vi "OpenSink.vi"(8 "error in (no error)":errorcluster, 11 "RelayAppender in":refnum<class "RelayAppender.lvclass">) -> (0 "error out":errorcluster, 3 "RelayAppender out":refnum<class "RelayAppender.lvclass">)   [LabVIEW 2026, in "Lumberjack.lvlib" / "RelayAppender.lvclass"]
doc: "Override of Appender.OpenSink, run once on actor startup. Queue mode: obtains the relay queue by its id-derived name (element type Statement) so the actor shares the same named queue the application holds, and stores the refnum in private data for Write to enqueue into. Message mode: validates the consumer enqueuer. Raises Lumberjack error +26 if the required resource is missing (queue not obtainable, or invalid enqueuer). Protected, dynamic-dispatch."
uses:
  RelayAppender.lvclass
  C:/Users/dallis/OneDrive - Velico Medical/Documents/Personal/LabVIEW Coding Projects/Lumberjack/src/Core/Appenders/Appender.lvclass/Appender.lvclass
  RelayAppender.lvclass/RelayAppender.ctl
  TypeDefs/Statement.ctl
  TypeDefs/Severity.ctl
  <vilib>/ActorFramework/Message Enqueuer/Message Enqueuer.lvclass
  Lumberjack.lvlib
  Appender.lvclass/Appender.lvclass
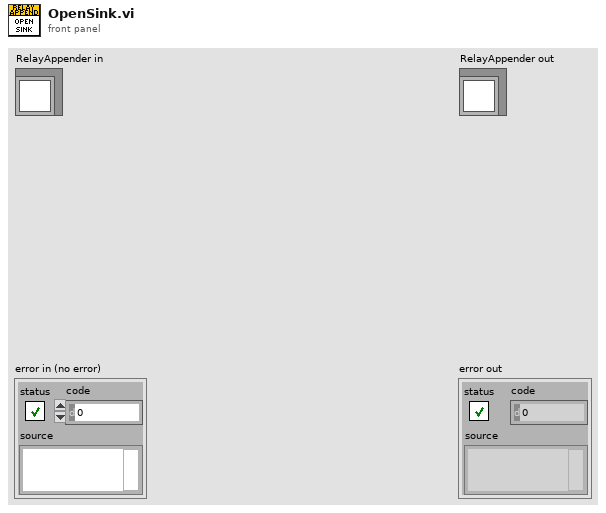
[diagram p1: front panel]
types:
  T1 = typedef "Lumberjack.lvlib/Statement.ctl" = cluster{"timestamp":timestamp, "level":T2, "sourceTag":string, "originVI":string, "message":string}
  T2 = typedef "Lumberjack.lvlib/Severity.ctl" = enum16{"OFF", "FATAL", "ERROR", "WARN", "INFO", "DEBUG", "TRACE", "ALL"}
  T3 = typedef "Lumberjack.lvlib/RelayMode.ctl" = enum16{"Message", "Queue"}
  T4 = typedef "Lumberjack.lvlib/AppenderConfig.ctl" = cluster{"id":string, "threshold":T2, "filter":T5, "queueBound":i32, "dropPolicy":T7, "useUTC":bool}
  T5 = typedef "Lumberjack.lvlib/Filter.ctl" = cluster{"mode":T6, "levelMin":T2, "levelMax":T2, "tagPrefix":string}
  T6 = typedef "Lumberjack.lvlib/FilterMode.ctl" = enum16{"Mirror", "Routed"}
  T7 = typedef "Lumberjack.lvlib/DropPolicy.ctl" = enum16{"DropOldest", "DropNewest", "LevelAware"}
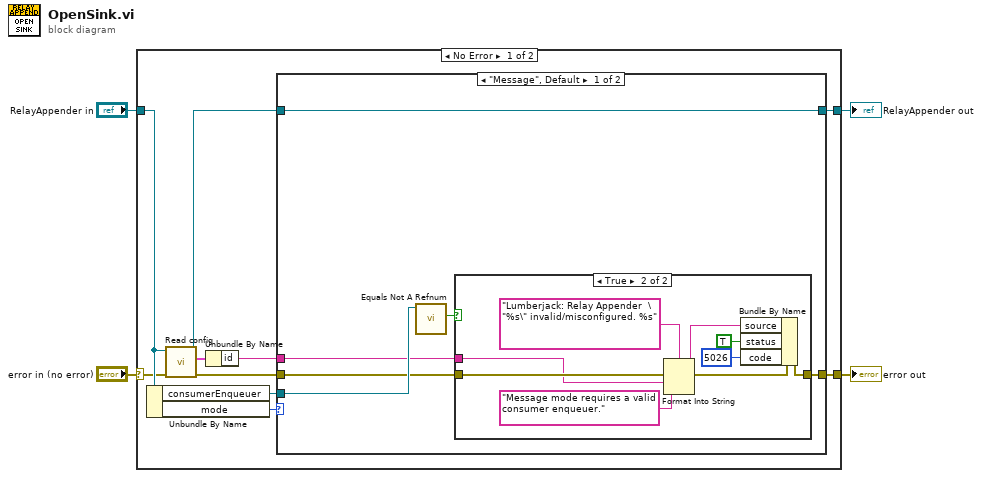
[diagram p0: block diagram]
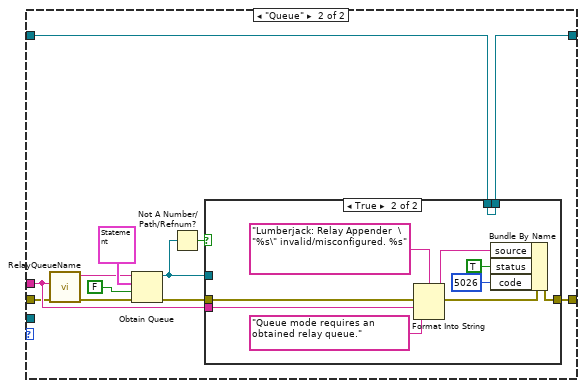
[diagram p3: hidden frame]
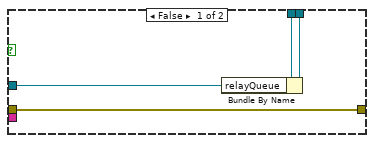
[diagram p4: hidden frame]
diagram:
  n1 = case shown="No Error" "error in (no error)" {
    selector: "error in (no error)" -> [w9 w58]
    tunnel: [w14 w58] -> w4
    tunnel: [w13 w57] -> w3
    tunnel: "RelayAppender in" -> [w10 w57]
    frame No Error {
      n2 = Unbundle By Name(w10) -> ("consumerEnqueuer"=w12:refnum<class "Message Enqueuer.lvclass">, "mode"=w11:T3)
      n3 = call "Read config.vi"("error in (no error)"=w9, "Appender in"=w10) -> ("error out"=w6:errorcluster, "AppenderConfig"=w8:T4, "Appender out"=w5:refnum<class "RelayAppender.lvclass">)  [unwired: 7 in]
      n4 = Unbundle By Name(w8) -> ("id"=w7:string)
      n5 = case shown="\"Message\", Default" w11 {
        tunnel: w12 -> [w20 _]
        tunnel: [w19 w42] -> w14
        tunnel: [w17 w37] -> w13
        tunnel: w7 -> [w15 w33]
        tunnel: w6 -> [w16 w32]
        tunnel: w5 -> [w17 w31]
        frame "Message", Default {
          n6 = call <vilib>:"Equals Not A Refnum.vi"("Message Enqueuer"=w20) -> ("Not a refnum?"=w18:bool)  [unwired: 10 in]
          n7 = case shown="True" w18 {
            tunnel: [w21 w25] -> w19
            tunnel: w16 -> [w21 w26]
            tunnel: w15 -> [_ w23]
            frame False {
            }
            frame True {
              n8 = Format Into String(format string="Lumberjack: Relay Appender  \"%s\" invalid/misconfigured. %s" ("source"), error in=w26, w23, "Message mode requires a valid consumer enqueuer.") -> (resulting string=w30:string, error out=w24:errorcluster)  [unwired: 1 in]
              n9 = Bundle By Name(cluster=w24, "source"=w30, "status"=TRUE, "code"=5026) -> (w25:errorcluster)
            }
          }
        }
        frame "Queue" {
          n10 = call "RelayQueueName.vi"("error in (no error)"=w32, "id"=w33) -> ("error out"=w35:errorcluster, "queueName"=w34:string)  [unwired: 8 in]
          n11 = Obtain Queue(name (unnamed)=w34, element data type=T1 {"timestamp"=timestamp(0 s since 1904-01-01), "level"=enum."INFO", "sourceTag"="", "originVI"="", "message"=""} ("Statement"), create if not found? (T)=FALSE, error in (no error)=w35) -> (queue out=w36:refnum<queue>, error out=w40:errorcluster)  [unwired: 1 in, 1 out]
          n12 = Not A Number/Path/Refnum?(number/path/refnum=w36) -> (NaN/Path/Refnum?=w41:bool)
          n13 = case shown="True" w41 {
            tunnel: [w46 w51] -> w42
            tunnel: w40 -> [w46 w52]
            tunnel: w33 -> [_ w50]
            tunnel: w31 -> [w45 w48]
            tunnel: [w44 w48] -> w37
            tunnel: w36 -> [w43 _]
            frame False {
              n14 = Bundle By Name(cluster=w45, "relayQueue"=w43) -> (w44:refnum<class "RelayAppender.lvclass">)
            }
            frame True {
              n15 = Format Into String(format string="Lumberjack: Relay Appender  \"%s\" invalid/misconfigured. %s" ("source"), error in=w52, w50, "Queue mode requires an obtained relay queue.") -> (resulting string=w56:string, error out=w49:errorcluster)  [unwired: 1 in]
              n16 = Bundle By Name(cluster=w49, "source"=w56, "status"=TRUE, "code"=5026) -> (w51:errorcluster)
            }
          }
        }
      }
    }
    frame Error {
    }
  }
  "error out" <- w4
  "RelayAppender out" <- w3
